vi "STR_Len.vi"() -> ()   [LabVIEW 2020]
panel:
  out "String 8":string
  out "String 6":string
  out "String 7":string
  in  "String 5":string
  in  "String 4":string
  out "Subset":string
  out "Concedenate":string
  in  "String 3":string
  in  "String 2":string
  out "Meter":u8(knob) scale=0.0..10.0
  in  "String":string
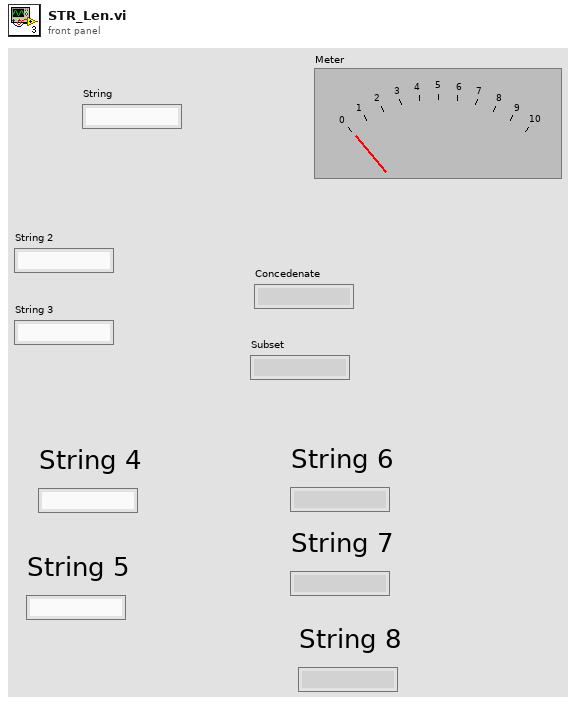
[diagram p1: front panel]
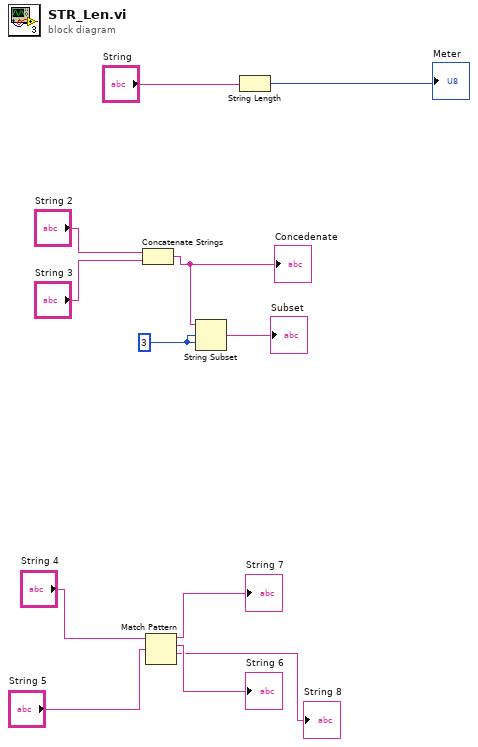
[diagram p0: block diagram]
diagram:
  w6 = 3
  n1 = Concatenate Strings("String 2", "String 3") -> (w8:string)
  "Concedenate" <- w8
  n2 = Match Pattern(string="String 4", regular expression="String 5") -> (before substring=→"String 7":string, match substring=→"String 6":string, after substring=→"String 8":string)  [unwired: 1 in, 1 out]
  n3 = String Subset(string=w8, offset (0)=w6, length (rest)=w6) -> (substring=→"Subset":string)
  n4 = String Length(string="String") -> (length=→"Meter":i32)
